vi "Initialize.vi"(8 "error in (no error)":errorcluster, 11 "VISA resource name":refnum<visa-resource-name>) -> (0 "error out":errorcluster, 3 "GE 5565PIORC":refnum<class "GE 5565PIORC.lvclass">)   [LabVIEW 2016, in "GE 5565PIORC.lvclass"]
uses:
  GE 5565PIORC.lvclass
  GE 5565PIORC.lvclass/GE 5565PIORC.ctl
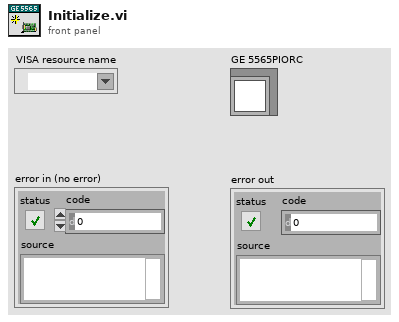
[diagram p1: front panel]
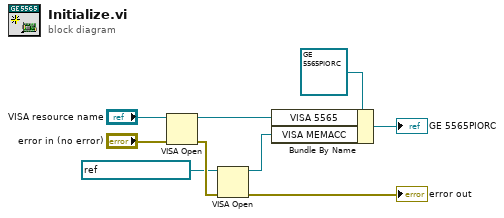
[diagram p0: block diagram]
diagram:
  n1 = VISA Open(error in (no error)="error in (no error)", VISA resource name="VISA resource name") -> (VISA resource name=w8:refnum<visa-resource-name>, error out=w4:errorcluster)  [unwired: 3 in]
  n2 = VISA Open(error in (no error)=w4, VISA resource name=refnum<visa-resource-name> "PXI0::MEMACC") -> (VISA resource name=w1:refnum<visa-resource-name>, error out=→"error out":errorcluster)  [unwired: 3 in]
  n3 = Bundle By Name(cluster=refnum<class "GE 5565PIORC.lvclass"> refnum ("GE 5565PIORC"), "VISA 5565"=w8, "VISA MEMACC"=w1) -> (→"GE 5565PIORC":refnum<class "GE 5565PIORC.lvclass">)
